vi "Pagina comandi manuali.vi"() -> (0 "pagina out":i16=255)   [LabVIEW 2022 SP3]
uses:
  <vilib>/Utility/miscctls.llb/LVKeyTypeDef.ctl
  Labview/Globali.vi
panel:
  out "CARRO IN POSIZIONE RP3000":bool
  out "CARRO IN POSIZIONE AAT":bool
  in  "Militare":bool
  out "VELOCITA' MOTORE":u16(knob) caption="Velocità \n[rpm]" scale=0.0..3000.0
  out "TEMPERATURA OLIO 10W30":sgl(slide) caption="Temperatura olio 10W30 [°C]" scale=0.0..100.0
  out "TEMPERATURA OLIO W90":sgl(slide) caption="Temperatura olio W90 [°C]" scale=0.0..100.0
  out "TEMPERATURA CUSCIN.":sgl(slide) caption="Temperatura\ncuscinetto\n[°C]" scale=0.0..120.0
  out "TEMPERATURA OLIO COPPA":sgl(slide) caption="Temperatura\nolio coppa\n[°C]" scale=0.0..120.0
  out "Trazione inserita":bool
  out "PRESSIONE RICIRCOLO":sgl(slide) caption="Pressione ricircolo [bar]" scale=0.0..2.5 scale format="%.1f"
  out "PORTATA RICIRCOLO":sgl(slide) caption="Portata ricircolo [l/min]" scale=0.0..25.0
  out "PRESSIONE ARIA 6 BAR":sgl(slide) caption="Pressione 6 bar [bar]" scale=0.0..10.0
  in  "Pagina parametri":bool
  out "Serial Number":string
  out "Prodotto":string
  out "PRESSURIZZAZIONE":sgl(slide) caption="Pressione pressurizz. [bar]" scale=0.0..1.0 scale format="%.1f"
  out "COPPIA ASSE":sgl(knob) caption="Coppia\n [Nm]" scale=0.0..100.0
  out "Erog. PROT35":bool
  in  "2. 3":bool
  out "Erog. W90":bool
  in  "2. 2":bool
  out "Erog. 10W30":bool
  in  "2. 1":bool
  out "Calibraz.tors.":bool
  in  "2. 5":bool
  out "Pompa PROT35":bool
  in  "2. 0":bool
  out "Pompa W90":bool
  in  "1. 7":bool
  out "Pompa 10W30":bool
  in  "1. 6":bool
  out "Scarico PROT35":bool
  in  "1. 3":bool
  out "Scarico W90":bool
  in  "1. 4":bool
  out "Scarico 10W30":bool
  in  "1. 5":bool
  out "Prova lampade":bool
  out "Pompa ricircolo":bool
  in  "1. 1":bool
  out "Ricircolo olio":bool
  in  "1. 2":bool
  out "Carico press.":bool
  in  "0. 7":bool
  out "Scarico press.":bool
  in  "1. 0":bool
  out "Scarico aria 6 bar":bool
  in  "0. 6":bool
  out "Carico aria 6 bar":bool
  in  "0. 5":bool
  out "S_MAN":bool
  in  "0. 0":bool
  out "S_AUTO":bool
  in  "0. 1":bool
  out "Rotaz.SX":bool
  in  "0. 2":bool
  out "Rotaz.DX":bool
  in  "0. 3":bool
  out "Start motore":bool
  in  "0. 4":bool
  in  "Vel.motore":i32(slide) min=0 max=3000 scale=0.0..3000.0
  out "Indicazioni":string
  in  "Prova":bool
  in  "Login":bool
  in  "stop":bool
  out "Comandi manuali":bool
  out "Tipo pagina":string
  out "Picture":picture
  out "Versione SW":dbl=1.0 format="%.2f"
  out "Linea":string="CENTAURO"
  in  "2. 4":bool
  out "TEMPERATURA AMBIENTE":sgl(slide) caption="Temperatura\nambiente\n[°C]" scale=0.0..50.0 scale format="%#.0f"
  out "Testo allarmi":string caption="ALLARMI"
  out "Testo fase collaudo":string caption="FASE COLLAUDO"
  out "Testo segnalazioni":string caption="SEGNALAZIONI"
  out "Testo messaggi":string caption="MESSAGGI"
  out "PLC->PC":string[](array[string])
  # "MOTORE"
  # "MODO FUNZIONAMENTO"
  # "CARICO/SCARICO ARIA"
  # "CARICO/SCARICO PRESSURIZZAZIONE"
  # "RICIRCOLO OLIO"
  # "OPERAZIONE"
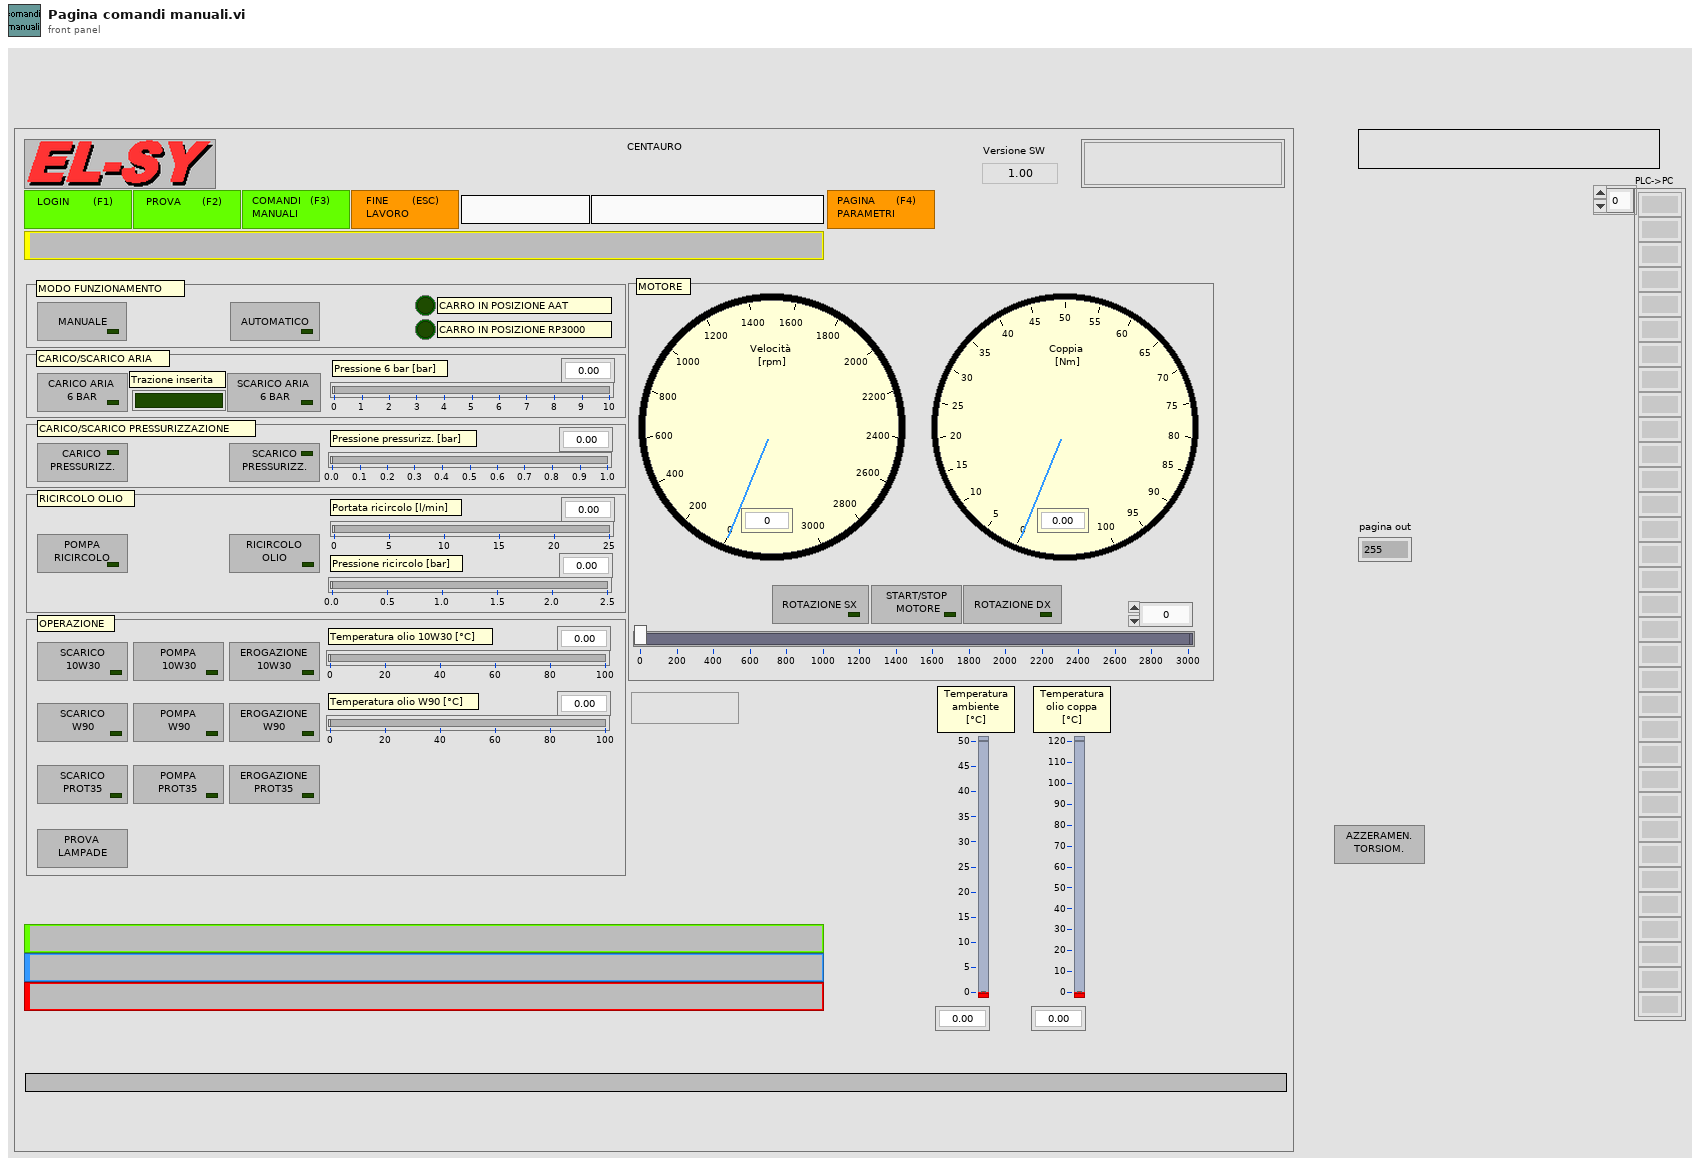
[diagram p1: front panel]
types:
  T1 = typedef "LVKeyTypeDef.ctl" = cluster{"Focus":bool, "Control":bool, "Shift":bool, "Key":string}
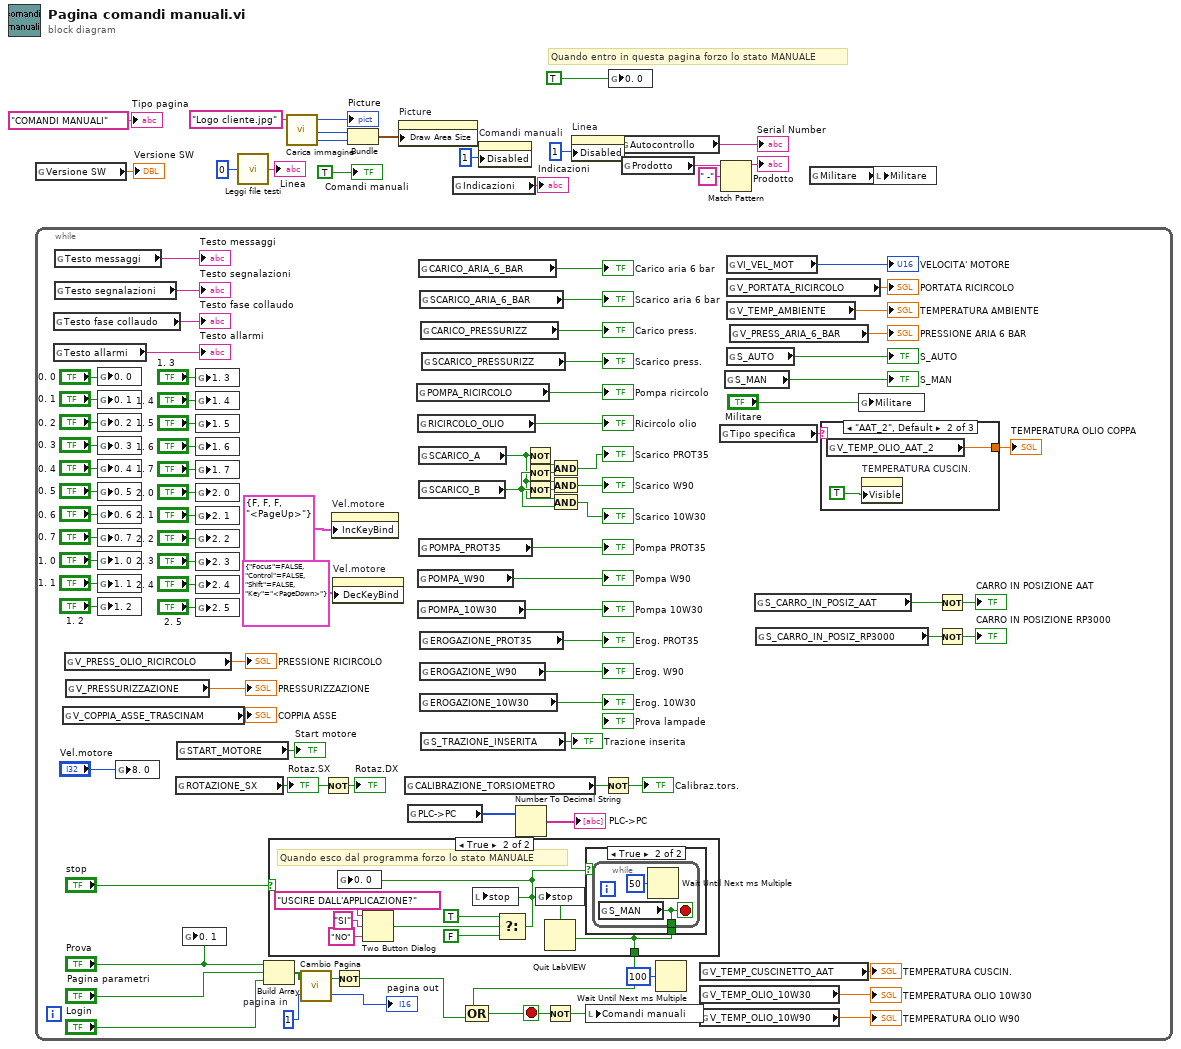
[diagram p0: block diagram]
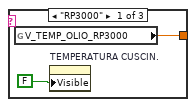
[diagram p2: hidden frame]
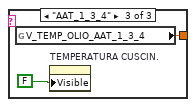
[diagram p3: hidden frame]
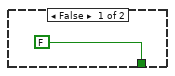
[diagram p4: hidden frame]
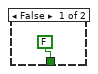
[diagram p5: hidden frame]
diagram:
  # "Quando entro in questa pagina forzo lo stato MANUALE"
  n1 = global read "globali.vi" "Versione SW"() -> (→"Versione SW":dbl)
  n2 = while {
    stop <- w92 stop-if-true
    w103 = u8 1  # pagina in
    n3 = global read "Globali.vi" "Testo fase collaudo"() -> (→"Testo fase collaudo":string)
    n4 = global read "Globali.vi" "Testo allarmi"() -> (→"Testo allarmi":string)
    n5 = global read "Globali.vi" "Testo messaggi"() -> (→"Testo messaggi":string)
    n6 = global read "Globali.vi" "Testo segnalazioni"() -> (→"Testo segnalazioni":string)
    n7 = global read "Globali.vi" "V_COPPIA_ASSE_TRASCINAM"() -> (→"COPPIA ASSE":sgl)
    n8 = global read "Globali.vi" "V_PRESS_OLIO_RICIRCOLO"() -> (→"PRESSIONE RICIRCOLO":sgl)
    n9 = global read "Globali.vi" "V_PRESSURIZZAZIONE"() -> (→"PRESSURIZZAZIONE":sgl)
    n10 = global write "Globali.vi" "0. 0"("0. 0") -> ()
    n11 = global write "Globali.vi" "0. 1"("0. 1") -> ()
    n12 = global write "Globali.vi" "0. 2"("0. 2") -> ()
    n13 = global write "Globali.vi" "0. 3"("0. 3") -> ()
    n14 = global write "Globali.vi" "0. 4"("0. 4") -> ()
    n15 = global write "Globali.vi" "0. 5"("0. 5") -> ()
    n16 = global write "Globali.vi" "0. 6"("0. 6") -> ()
    n17 = global write "Globali.vi" "0. 7"("0. 7") -> ()
    n18 = global write "Globali.vi" "1. 0"("1. 0") -> ()
    n19 = global write "Globali.vi" "1. 1"("1. 1") -> ()
    n20 = global write "Globali.vi" "1. 2"("1. 2") -> ()
    n21 = global write "Globali.vi" "8. 0"("Vel.motore") -> ()
    n22 = global read "Globali.vi" "ROTAZIONE_SX"() -> (w63:bool)
    "Rotaz.SX" <- w63
    n23 = global read "Globali.vi" "START_MOTORE"() -> (→"Start motore":bool)
    n24 = global write "Globali.vi" "0. 1"("Prova") -> ()
    n25 = global write "Globali.vi" "1. 3"("1. 3") -> ()
    n26 = global write "Globali.vi" "1. 4"("1. 4") -> ()
    n27 = global write "Globali.vi" "1. 5"("1. 5") -> ()
    n28 = global write "Globali.vi" "1. 6"("1. 6") -> ()
    n29 = global write "Globali.vi" "1. 7"("1. 7") -> ()
    n30 = global write "Globali.vi" "2. 0"("2. 0") -> ()
    n31 = global write "Globali.vi" "2. 1"("2. 1") -> ()
    n32 = global write "Globali.vi" "2. 2"("2. 2") -> ()
    n33 = global write "Globali.vi" "2. 3"("2. 3") -> ()
    n34 = global write "Globali.vi" "2. 4"("2. 4") -> ()
    n35 = global write "Globali.vi" "2. 5"("2. 5") -> ()
    n36 = Build Array("Prova", "Pagina parametri", "Login") -> (w102:bool[])
    n37 = case shown="True" "stop" {
      tunnel: [FALSE ("x = y?") w117] -> w88
      frame False {
      }
      frame True {
        # "Quando esco dal programma forzo lo stato MANUALE"
        n38 = Two Button Dialog(message="USCIRE DALL'APPLICAZIONE?" ("T button name (\"OK\")"), 1:"NO" ("F button name (\"Cancel\")"), 2:"SI" ("T button name (\"OK\")")) -> (T button?=w122:bool)
        n39 = Select(t=TRUE, s=w122, f=FALSE) -> (s? t:f=w116:bool)
        n40 = global write "Globali.vi" "0. 0"(w116) -> ()
        n41 = local write "stop"(w116) -> ()
        n42 = case shown="True" w116 {
          tunnel: [FALSE ("S_MAN") w125] -> w117
          frame False {
          }
          frame True {
            n43 = while {
              tunnel: [w126] -> w125
              stop <- w126 stop-if-true
              n44 = global read "Globali.vi" "S_MAN"() -> (w126:bool)
              n45 = Wait Until Next ms Multiple(millisecond multiple=u32 50) -> ()  [unwired: 1 out]
            }
          }
        }
        n46 = global write "Globali.vi" "stop"(w117) -> ()
        n47 = Quit LabVIEW(quit? (T)=w117) -> ()
      }
    }
    n48 = call "Cambio Pagina.vi"("pagina in"=w103, "pulsanti"=w102) -> ("pagina out"=→"pagina out":u8, "premuto"=w105:bool)
    n49 = Not(x=w63) -> (.not. x?=→"Rotaz.DX":bool)
    n50 = property on="Vel.motore" class="Slide (strict)"("IncKeyBind"=T1 {"Focus"=FALSE, "Control"=FALSE, "Shift"=FALSE, "Key"="<PageUp>"} ("Increment Key Binding")) -> ()  [unwired: 2 in, 2 out]
    n51 = property on="Vel.motore" class="Slide (strict)"("DecKeyBind"=T1 {"Focus"=FALSE, "Control"=FALSE, "Shift"=FALSE, "Key"="<PageDown>"} ("Decrement Key Binding")) -> ()  [unwired: 2 in, 2 out]
    n52 = Not(x=w105) -> (.not. x?=w101:bool)
    n53 = global read "Globali.vi" "CALIBRAZIONE_TORSIOMETRO"() -> (w40:bool)
    n54 = global read "Globali.vi" "PLC->PC"() -> (w107:u16[])
    n55 = global read "Globali.vi" "POMPA_RICIRCOLO"() -> (→"Pompa ricircolo":bool)
    n56 = global read "Globali.vi" "RICIRCOLO_OLIO"() -> (→"Ricircolo olio":bool)
    n57 = global read "Globali.vi" "POMPA_W90"() -> (→"Pompa W90":bool)
    n58 = global read "Globali.vi" "POMPA_10W30"() -> (→"Pompa 10W30":bool)
    n59 = global read "Globali.vi" "CARICO_ARIA_6_BAR"() -> (→"Carico aria 6 bar":bool)
    n60 = global read "Globali.vi" "SCARICO_A"() -> (w54:bool)
    n61 = global read "Globali.vi" "SCARICO_B"() -> (w55:bool)
    n62 = global read "Globali.vi" "POMPA_PROT35"() -> (→"Pompa PROT35":bool)
    n63 = global read "Globali.vi" "SCARICO_ARIA_6_BAR"() -> (→"Scarico aria 6 bar":bool)
    n64 = global read "Globali.vi" "EROGAZIONE_PROT35"() -> (→"Erog. PROT35":bool)
    n65 = global read "Globali.vi" "EROGAZIONE_W90"() -> (→"Erog. W90":bool)
    n66 = global read "Globali.vi" "EROGAZIONE_10W30"() -> (→"Erog. 10W30":bool)
    n67 = global read "Globali.vi" "CARICO_PRESSURIZZ"() -> (→"Carico press.":bool)
    n68 = global read "Globali.vi" "S_TRAZIONE_INSERITA"() -> (→"Trazione inserita":bool)
    n69 = global read "Globali.vi" "SCARICO_PRESSURIZZ"() -> (→"Scarico press.":bool)
    n70 = Compound Arithmetic op=OR(w88, w101) -> (w92:bool)
    n71 = Number To Decimal String(number=w107) -> (decimal integer string=→"PLC->PC":string[])  [unwired: 1 in]
    n72 = Not(x=w54) -> (.not. x?=w51:bool)
    n73 = Not(x=w55) -> (.not. x?=w52:bool)
    n74 = Not(x=w55) -> (.not. x?=w53:bool)
    n75 = Not(x=w92) -> (.not. x?=w91:bool)
    n76 = And(x=w51, y=w52) -> (x .and. y?=→"Scarico PROT35":bool)
    n77 = And(x=w54, y=w53) -> (x .and. y?=→"Scarico W90":bool)
    n78 = And(x=w54, y=w55) -> (x .and. y?=→"Scarico 10W30":bool)
    n79 = local write "Comandi manuali"(w91) -> ()
    n80 = Not(x=w40) -> (.not. x?=→"Calibraz.tors.":bool)
    n81 = Wait Until Next ms Multiple(millisecond multiple=u32 100) -> ()  [unwired: 1 out]
    n82 = global read "Globali.vi" "V_TEMP_CUSCINETTO_AAT"() -> (→"TEMPERATURA CUSCIN.":sgl)
    n83 = global read "Globali.vi" "V_TEMP_OLIO_10W30"() -> (→"TEMPERATURA OLIO 10W30":sgl)
    n84 = global read "Globali.vi" "V_TEMP_OLIO_10W90"() -> (→"TEMPERATURA OLIO W90":sgl)
    n85 = global read "Globali.vi" "Tipo specifica"() -> (w29:string)
    n86 = global read "Globali.vi" "S_MAN"() -> (→"S_MAN":bool)
    n87 = global read "Globali.vi" "VI_VEL_MOT"() -> (→"VELOCITA' MOTORE":u16)
    n88 = global read "Globali.vi" "V_PORTATA_RICIRCOLO"() -> (→"PORTATA RICIRCOLO":sgl)
    n89 = global read "Globali.vi" "V_TEMP_AMBIENTE"() -> (→"TEMPERATURA AMBIENTE":sgl)
    n90 = global read "Globali.vi" "S_AUTO"() -> (→"S_AUTO":bool)
    n91 = global read "Globali.vi" "V_PRESS_ARIA_6_BAR"() -> (→"PRESSIONE ARIA 6 BAR":sgl)
    n92 = global read "Globali.vi" "S_CARRO_IN_POSIZ_AAT"() -> (w23:bool)
    n93 = global read "Globali.vi" "S_CARRO_IN_POSIZ_RP3000"() -> (w22:bool)
    n94 = case shown="\"AAT_2\", Default" w29 {
      tunnel: [w110 w112 w114] -> w31
      frame "RP3000" {
        n95 = global read "Globali.vi" "V_TEMP_OLIO_RP3000"() -> (w110:sgl)
        n96 = property on="TEMPERATURA CUSCIN." class="Slide (strict)"("Visible"=FALSE) -> ()  [unwired: 2 in, 2 out]
      }
      frame "AAT_2", Default {
        n97 = global read "Globali.vi" "V_TEMP_OLIO_AAT_2"() -> (w112:sgl)
        n98 = property on="TEMPERATURA CUSCIN." class="Slide (strict)"("Visible"=TRUE) -> ()  [unwired: 2 in, 2 out]
      }
      frame "AAT_1_3_4" {
        n99 = global read "Globali.vi" "V_TEMP_OLIO_AAT_1_3_4"() -> (w114:sgl)
        n100 = property on="TEMPERATURA CUSCIN." class="Slide (strict)"("Visible"=FALSE) -> ()  [unwired: 2 in, 2 out]
      }
    }
    "TEMPERATURA OLIO COPPA" <- w31
    n101 = global write "Globali.vi" "Militare"("Militare") -> ()
    n102 = Not(x=w23) -> (.not. x?=→"CARRO IN POSIZIONE AAT":bool)
    n103 = Not(x=w22) -> (.not. x?=→"CARRO IN POSIZIONE RP3000":bool)
  }
  n104 = call "Leggi file testi.vi"("Numero riga"=0) -> ("Testo"=→"Linea":string)  [unwired: 3 in, 1 out]
  n105 = call "Carica immagine.vi"("Immagine JPG"="Logo cliente.jpg") -> ("altezza"=w15:i16, "larghezza"=w16:i16, "Picture"=→"Picture":picture)  [unwired: 2 in]
  n106 = Bundle("larghezza"=w16, "altezza"=w15) -> (w14:cluster{"larghezza":i16, "altezza":i16})  [unwired: 1 in]
  n107 = property on="Picture" class="Pict"("Draw Area Size"=w14) -> ()  [unwired: 2 in, 2 out]
  n108 = global read "Globali.vi" "Indicazioni"() -> (→"Indicazioni":string)
  n109 = property on="Comandi manuali" class="Bool"("Disabled"=u8 1) -> ()  [unwired: 2 in, 2 out]
  n110 = property on="Linea" class="Str"("Disabled"=u8 1) -> ()  [unwired: 2 in, 2 out]
  n111 = global write "Globali.vi" "0. 0"(TRUE ("0. 0")) -> ()
  n112 = global read "Globali.vi" "Autocontrollo"() -> (→"Serial Number":string)
  n113 = global read "Globali.vi" "Prodotto"() -> (w5:string)
  n114 = Match Pattern(string=w5, regular expression=" -") -> (before substring=→"Prodotto":string)  [unwired: 1 in, 3 out]
  n115 = global read "Globali.vi" "Militare"() -> (w1:bool)
  n116 = local write "Militare"(w1) -> ()
  "Tipo pagina" <- "COMANDI MANUALI" ("Tipo pagina")
  "Comandi manuali" <- TRUE ("Comandi manuali")
